vi "fgv_NtripGNSS_process-val.vi"(7 "cmd":T2, 11 "process val":T1={"GNSS time"="", "Ntrip conn"=FALSE, "NMEA val"=FALSE, "ycenter_TM"=0.0, "xcenter_TM"=0.0, "TM ref circles"=[], "RTCM recv-str"="", "GNSS Serail buff N"=0, "Sel NMEA type"=enum."$GPGGA", "RTCM recv_sourcetable"="", "NMEA cluster"={"GxGGA"="", "GxGSV"="", "GNRMC"="", "GxTXT"="", "GxGSA"="", "GxGLL"=""}, "Sel NMEA str"="", "NMEA recv-str"=""}) -> (3 "process val out":T1={"GNSS time"="", "Ntrip conn"=FALSE, "NMEA val"=FALSE, "ycenter_TM"=0.0, "xcenter_TM"=0.0, "TM ref circles"=[], "RTCM recv-str"="", "GNSS Serail buff N"=0, "Sel NMEA type"=enum."$GPGGA", "RTCM recv_sourcetable"="", "NMEA cluster"={"GxGGA"="", "GxGSV"="", "GNRMC"="", "GxTXT"="", "GxGSA"="", "GxGLL"=""}, "Sel NMEA str"="", "NMEA recv-str"=""})   [LabVIEW 2019]
uses:
  Ctrl/cmd_ini-RW.ctl
  Ctrl/GNSS-Ntrip process val.ctl
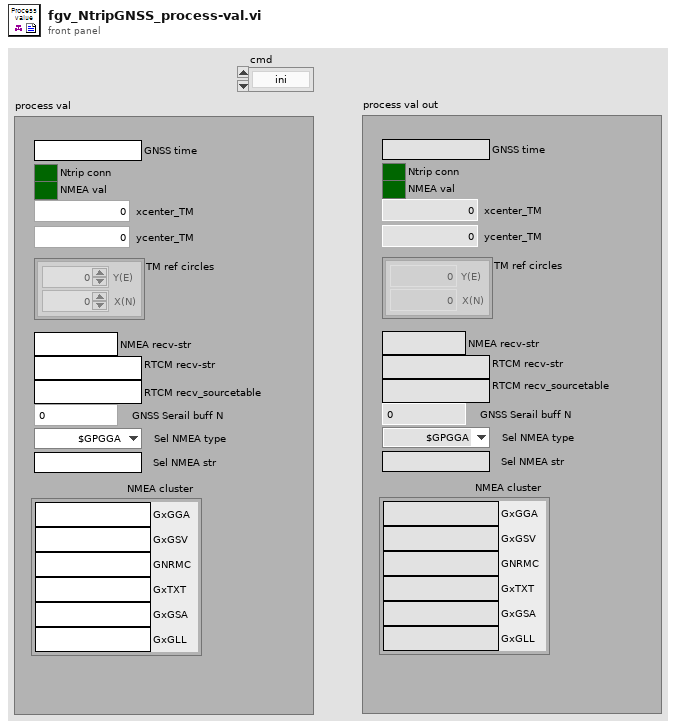
[diagram p1: front panel]
types:
  T1 = typedef "GNSS-Ntrip process val.ctl" = cluster{"GNSS time":string, "Ntrip conn":bool, "NMEA val":bool, "ycenter_TM":dbl, "xcenter_TM":dbl, "TM ref circles":cluster{"Y(E)":dbl, "X(N)":dbl}[], "RTCM recv-str":string, "GNSS Serail buff N":u32, "Sel NMEA type":enum16{"$GPGSV", "$GLGSV", "$GPGGA", "$GAGSV", "$GBGSV", "$GNGLL", "$GNGGA", "$GNGSA", "$GNRMC", "$GNVTG"}, "RTCM recv_sourcetable":string, "NMEA cluster":cluster{"GxGGA":string, "GxGSV":string, "GNRMC":string, "GxTXT":string, "GxGSA":string, "GxGLL":string}, "Sel NMEA str":string, "NMEA recv-str":string}
  T2 = typedef "cmd_ini-RW.ctl" = enum16{"ini", "read", "write"}
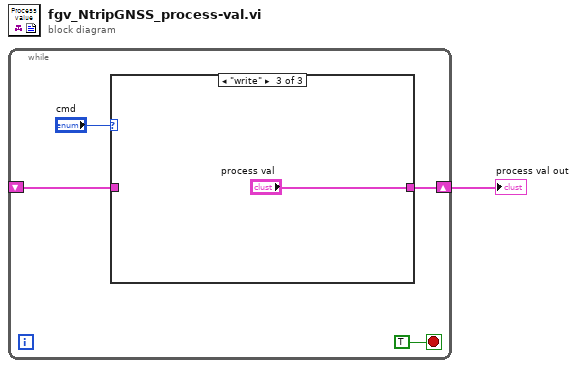
[diagram p0: block diagram]
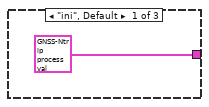
[diagram p2: hidden frame]
diagram:
  n1 = while {
    shift-right: [w3] -> w1
    shift-left: _ -> [w2]
    stop <- TRUE stop-if-true
    n2 = case shown="\"write\"" "cmd" {
      tunnel: [T1 {"GNSS time"="", "Ntrip conn"=TRUE, "NMEA val"=FALSE, "ycenter_TM"=532752.4315145966, "xcenter_TM"=195466.20176298777, "TM ref circles"=[], "RTCM recv-str"="", "GNSS Serail buff N"=0, "Sel NMEA type"=enum."$GPGGA", "RTCM recv_sourcetable"="", "NMEA cluster"={"GxGGA"="", "GxGSV"="", "GNRMC"="", "GxTXT"="", "GxGSA"="", "GxGLL"=""}, "Sel NMEA str"="", "NMEA recv-str"=""} ("process val") w7 "process val"] -> w3
      tunnel: w2 -> [_ w7 _]
      frame "ini", Default {
      }
      frame "read" {
      }
      frame "write" {
      }
    }
  }
  "process val out" <- w1
